vi "initialize_log.vi"(8 "error in (no error)":errorcluster, 10 "swabian_local_data 3":T1={"events"={"update_status"=refnum, "update_chart"=refnum, "update_xy"=refnum, "send_channel_data"=refnum}, "stop_q"=refnum, "tagger_reference"=refnum, "connect_button"=refnum, "counter_reference"=refnum, "tagger_stream_reference"=refnum, "log_reference"=refnum, "current_log_offset"=0, "tt20_buffer_q"=refnum, "stream_to_file_button"=refnum, "num_records"=0, "connected?"=FALSE, "plots"=refnum, "histogram_bin_edges"=[], "histogrammer"=refnum, "plot_lifetimes"=refnum, "xy_graph"=refnum, "Reference\nChannel"=enum."ch0", "trigger_channels"=[], "filter_channels"=[], "active_channels"=[], "acq_mode"=0, "Reference\nChannel"=enum."ch0", "acq_time"=0, "leftovers"={"leftover_stamps"=[], "leftover_channels"=[], "any?"=FALSE}, "sync_period_ps"=0, "raw_stream_path"=path "", "Leftovers"={"missing_sync_data"=[], "missing_events"=0}, "first_batch"=0, "first_sync_stamp"=0, "lifetime_settings"={"Plot Lifetimes"=FALSE, "start_time"=0.0, "stop_time"=0.0, "n_bins"=0}, "Histogram_bins"=[], "last_processed_data"=[], "histogram_data"=[]}, 11 "Data_path":path) -> (0 "error out":errorcluster, 3 "swabian_local_data 2":T1={"events"={"update_status"=refnum, "update_chart"=refnum, "update_xy"=refnum, "send_channel_data"=refnum}, "stop_q"=refnum, "tagger_reference"=refnum, "connect_button"=refnum, "counter_reference"=refnum, "tagger_stream_reference"=refnum, "log_reference"=refnum, "current_log_offset"=0, "tt20_buffer_q"=refnum, "stream_to_file_button"=refnum, "num_records"=0, "connected?"=FALSE, "plots"=refnum, "histogram_bin_edges"=[], "histogrammer"=refnum, "plot_lifetimes"=refnum, "xy_graph"=refnum, "Reference\nChannel"=enum."ch0", "trigger_channels"=[], "filter_channels"=[], "active_channels"=[], "acq_mode"=0, "Reference\nChannel"=enum."ch0", "acq_time"=0, "leftovers"={"leftover_stamps"=[], "leftover_channels"=[], "any?"=FALSE}, "sync_period_ps"=0, "raw_stream_path"=path "", "Leftovers"={"missing_sync_data"=[], "missing_events"=0}, "first_batch"=0, "first_sync_stamp"=0, "lifetime_settings"={"Plot Lifetimes"=FALSE, "start_time"=0.0, "stop_time"=0.0, "n_bins"=0}, "Histogram_bins"=[], "last_processed_data"=[], "histogram_data"=[]})   [LabVIEW 2018]
uses:
  swabian_local_data_tdef.ctl
  swabian_events_tdef.ctl
  update_chart_tdef.ctl
  channel_data_tdef.ctl
  C:/Users/bspoka/Documents/swabian_LV/lib/TTCSharp32.dll
  lib/TTCSharp32.dll
  swabian_buffer_tdef.ctl
  reference_checkbox_tdef.ctl
  leftovers_struct.ctl
  lifetime_settings.ctl
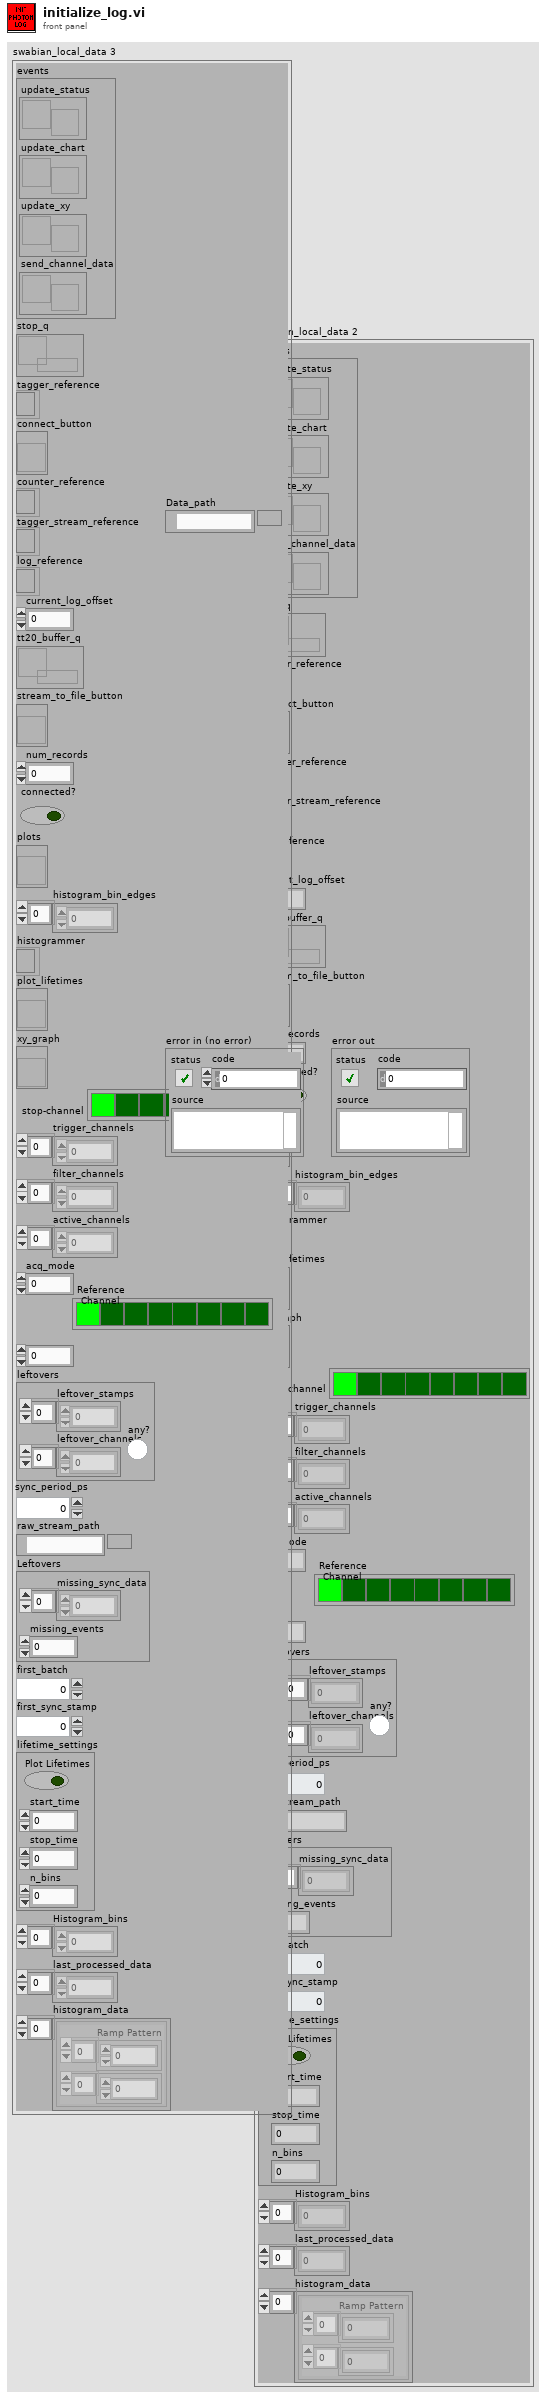
[diagram p1: front panel]
types:
  T1 = typedef "swabian_local_data_tdef.ctl" = cluster{"events":T2, "stop_q":refnum<queue>, "tagger_reference":refnum<k24>, "connect_button":refnum<vi>, "counter_reference":refnum<k24>, "tagger_stream_reference":refnum<k24>, "log_reference":refnum<file>, "current_log_offset":i64, "tt20_buffer_q":refnum<queue>, "stream_to_file_button":refnum<vi>, "num_records":u64, "connected?":bool, "plots":refnum<vi>, "histogram_bin_edges":i64[], "histogrammer":refnum<k24>, "plot_lifetimes":refnum<vi>, "xy_graph":refnum<vi>, "Reference\nChannel":T3, "trigger_channels":i32[], "filter_channels":i32[], "active_channels":i32[], "acq_mode":i32, "Reference\nChannel":T3, "acq_time":i64, "leftovers":T4, "sync_period_ps":i64, "raw_stream_path":path, "Leftovers":cluster{"missing_sync_data":u64[], "missing_events":i32}, "first_batch":i32, "first_sync_stamp":u64, "lifetime_settings":T5, "Histogram_bins":dbl[], "last_processed_data":u64[], "histogram_data":cluster{"Ramp Pattern":dbl[], dbl[]}[]}
  T2 = typedef "swabian_events_tdef.ctl" = cluster{"update_status":refnum<user-event>, "update_chart":refnum<user-event>, "update_xy":refnum<user-event>, "send_channel_data":refnum<user-event>}
  T3 = typedef "reference_checkbox_tdef.ctl" = enum32{"No Selection", "ch0", "ch1", "ch2", "ch3", "ch4", "ch5", "ch6", "ch7"}
  T4 = typedef "leftovers_struct.ctl" = cluster{"leftover_stamps":i64[], "leftover_channels":i32[], "any?":bool}
  T5 = typedef "lifetime_settings.ctl" = cluster{"Plot Lifetimes":bool, "start_time":dbl, "stop_time":dbl, "n_bins":i32}
  T6 = enum16{"open", "replace", "create", "open or create", "replace or create", "replace or create with confirmation"}
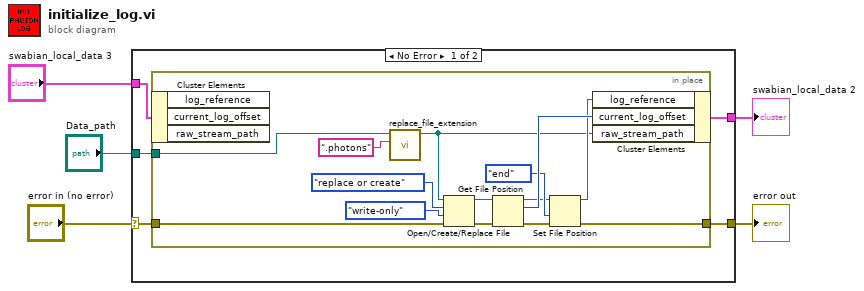
[diagram p0: block diagram]
diagram:
  n1 = case shown="No Error" "error in (no error)" {
    selector: "error in (no error)" -> [w6 w25]
    tunnel: [w10 w26] -> w5
    tunnel: "swabian_local_data 3" -> [w9 w26]
    tunnel: [w8 w25] -> w3
    tunnel: "Data_path" -> [w7 _]
    frame No Error {
      n2 = in-place {
        in-place-border: w7 -> [w13]
        in-place-border: w6 -> [w22]
        in-place-border: [w16] -> w8
        n3 = in-place-cluster #1(w9) -> ()  [unwired: 3 out]
        n4 = call "replace_file_extension.vi"("new_extension"=".photons", "data_path"=w13) -> ("appended path"=w11:path)  [unwired: 8 in, 1 out]
        n5 = Open/Create/Replace File(file path (use dialog)=w11, error in=w22, operation (0:open)=T6."replace or create", access (0:read/write)=enum16{"read/write", "read-only", "write-only"}."write-only") -> (refnum out=w20:refnum<file>, error out=w21:errorcluster)  [unwired: 2 in, 1 out]
        n6 = Get File Position(4:w21, 7:w20) -> (0:w17:errorcluster, 2:w19:i64, 3:w15:refnum<file>)
        n7 = Set File Position(refnum=w15, from (0:start)=enum16{"start", "end", "current"}."end", error in=w17) -> (refnum out=w14:refnum<file>, error out=w16:errorcluster)  [unwired: 1 in]
        n8 = in-place-cluster #1("log_reference"=w14, "current_log_offset"=w19, "raw_stream_path"=w11) -> (w10:T1)
      }
    }
    frame Error {
    }
  }
  "swabian_local_data 2" <- w5
  "error out" <- w3
